vi "ConfigureAdaptorr00.vi"() -> ()   [LabVIEW 2011]
panel:
  out "error out":errorcluster
  out "concatenated string":string
  in  "Trip Point 1(Torr)":dbl=700.0
  in  "Set Point D (Torr)":dbl=40.0
  in  "Set Point C (Torr)":dbl=20.0
  in  "Set Point B (Torr)":dbl=76.0
  in  "Set Point A (Torr)":dbl=10.0
  in  "Trip Point 2 (Torr)":dbl=200.0
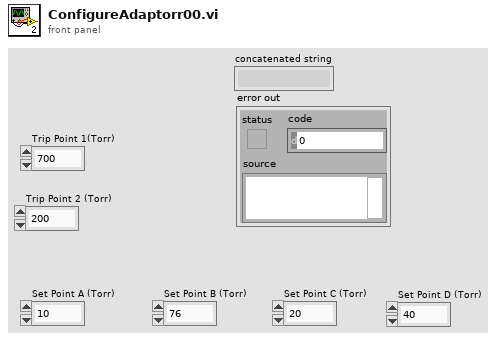
[diagram p1: front panel]
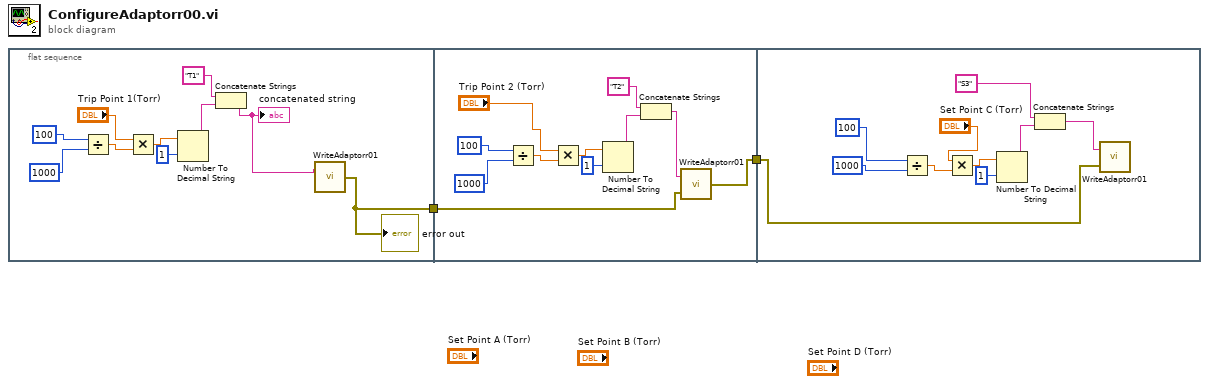
[diagram p0: block diagram]
diagram:
  n1 = flat-sequence {
    tunnel: [w3] -> w1
    tunnel: [w13] -> w2
    tunnel: w1 -> [w15]
    tunnel: w2 -> [w24]
    frame #0 {
      n2 = Divide(x=100, y=1000) -> (x/y=w10:dbl)
      n3 = Multiply(x="Trip Point 1(Torr)", y=w10) -> (x*y=w8:dbl)
      n4 = Number To Decimal String(number=w8, width (-)=i16 1) -> (decimal integer string=w5:string)
      n5 = Concatenate Strings("T1", w5) -> (w4:string)
      "concatenated string" <- w4
      n6 = call "WriteAdaptorr01.vi"("string to write"=w4) -> ("error out"=w3:errorcluster)  [unwired: 1 in]
      "error out" <- w3
    }
    frame #1 {
      n7 = Divide(x=100, y=1000) -> (x/y=w21:dbl)
      n8 = Multiply(x="Trip Point 2 (Torr)", y=w21) -> (x*y=w20:dbl)
      n9 = Number To Decimal String(number=w20, width (-)=i16 1) -> (decimal integer string=w17:string)
      n10 = Concatenate Strings("T2", w17) -> (w14:string)
      n11 = call "WriteAdaptorr01.vi"("error in (no error)"=w15, "string to write"=w14) -> ("error out"=w13:errorcluster)
    }
    frame #2 {
      n12 = Divide(x=100, y=1000) -> (x/y=w31:dbl)
      n13 = Multiply(x="Set Point C (Torr)", y=w31) -> (x*y=w28:dbl)
      n14 = Number To Decimal String(number=w28, width (-)=i16 1) -> (decimal integer string=w26:string)
      n15 = Concatenate Strings("S3", w26) -> (w25:string)
      n16 = call "WriteAdaptorr01.vi"("error in (no error)"=w24, "string to write"=w25) -> ()  [unwired: 1 out]
    }
  }
